vi "CameraGetData.vi"(8 "error in (no error)":errorcluster, 10 "keep open?":bool, 11 "NIvision in":refnum<class "IMAQdx.lvclass">) -> (0 "error out":errorcluster, 2 "image_data":u16[][][](array[numeric]), 3 "NIvision out":refnum<class "IMAQdx.lvclass">)   [LabVIEW 2010, in "IMAQdx.lvclass"]
uses:
  <userlib>/BIAS2/classes/IMAQdx/IMAQdx.lvclass
  <userlib>/BIAS2/classes/IMAQdx/IMAQdx.lvclass/IMAQdx.ctl
  <vilib>/vision/driver/IMAQdx.llb/IMAQdx Buffer Number Mode.ctl
  <vilib>/vision/driver/NI_Vision_Acquisition_Software.lvlib
  resource/objmgr/imaqdx.rc
  <userlib>/BIAS2/c/imaging_tools.dll
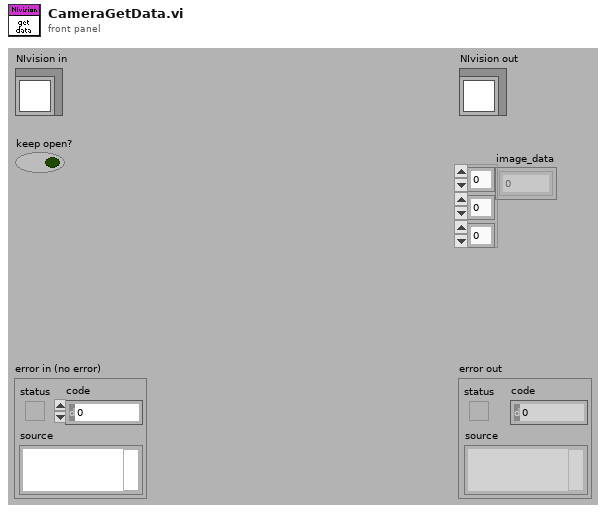
[diagram p1: front panel]
types:
  T1 = typedef "NI_Vision_Acquisition_Software.lvlib/IMAQdx Buffer Number Mode.ctl" = enum32{"Next", "Last", "Buffer Number"}
  T2 = typedef "IMAQdx.ctl" = refnum<k21>
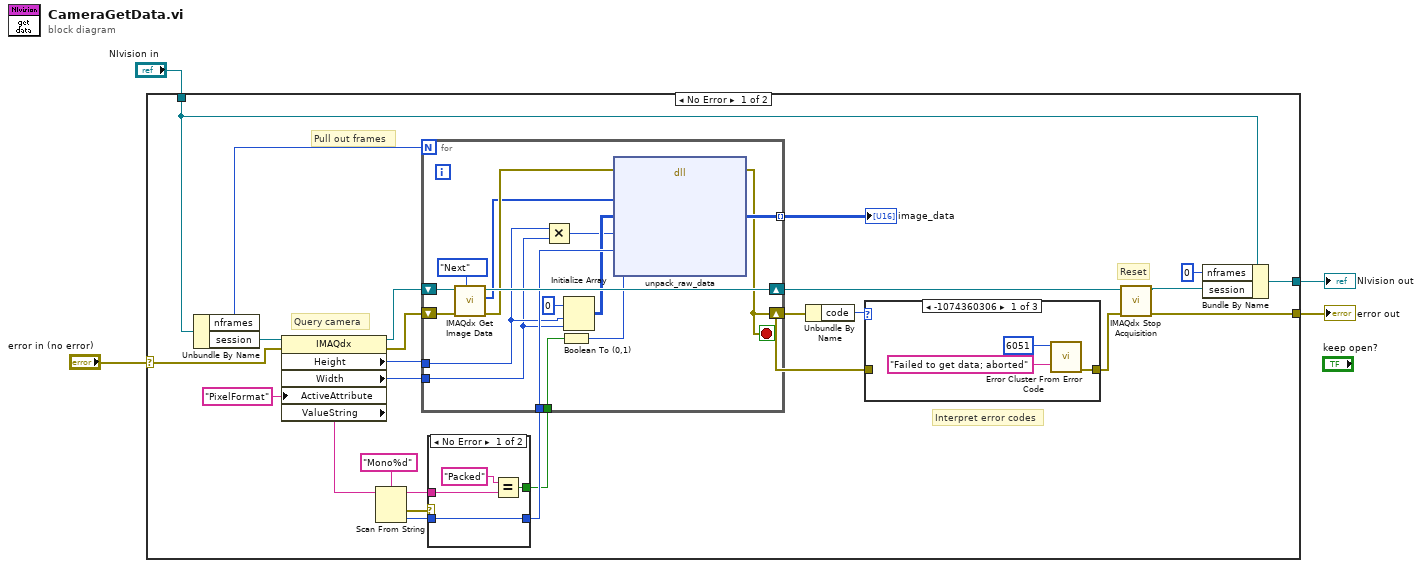
[diagram p0: block diagram]
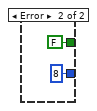
[diagram p2: hidden frame]
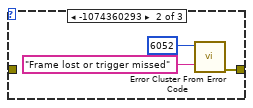
[diagram p3: hidden frame]
diagram:
  n1 = case shown="No Error" "error in (no error)" {
    selector: "error in (no error)" -> [w10 w59]
    tunnel: "NIvision in" -> [w25 w60]
    tunnel: [w9 w60] -> w2
    tunnel: [w7 w59] -> w1
    frame No Error {
      # "Query camera"
      # "Interpret error codes"
      # "Reset"
      # "Pull out frames"
      n2 = Unbundle By Name(w25) -> ("nframes"=w24:i32, "session"=w6:refnum<k21>)
      n3 = property class="IMAQdx"(reference=w6, error in=w10, "ActiveAttribute"="PixelFormat") -> (reference out=w5:refnum<k21>, error out=w28:errorcluster, "Height"=w27:u32, "Width"=w26:u32, "ValueString"=w17:string)
      n4 = Scan From String(format string="Mono%d", input string=w17) -> (remaining string=w16:string, error out=w15:errorcluster, output 1=w14:i32)  [unwired: 3 in, 1 out]
      n5 = case shown="No Error" w15 {
        tunnel: w16 -> [w33 _]
        tunnel: [w31 FALSE] -> w12
        tunnel: [w30 8] -> w13
        tunnel: w14 -> [w30 _]
        frame No Error {
          n6 = Equal?(x="Packed" ("format string"), y=w33) -> (x = y?=w31:bool)
        }
        frame Error {
        }
      }
      n7 = for {
        N: w24 -> [_]
        tunnel: [w53] -> w11 mode=indexing
        shift-right: [w57] -> w29
        shift-left: w5 -> [w58]
        shift-right: [w43] -> w21
        shift-left: w28 -> [w56]
        tunnel: w27 -> [w52]
        tunnel: w26 -> [w51]
        tunnel: w13 -> [w55]
        tunnel: w12 -> [w54]
        stop <- w43 stop-if-true
        n8 = call <vilib>:"IMAQdx Get Image Data.vi"("Buffer Number Mode (Next)"=IMAQdx_Buffer_Number_Mode."Next", "error in"=w56, "Session In"=w58) -> ("error out"=w45:errorcluster, "Image Data Array"=w44:u8[], "Session Out"=w57:T2)  [unwired: 5 in, 1 out]
        n9 = Multiply(x=w52, y=w51) -> (x*y=w47:u32)
        n10 = Boolean To (0,1)(Boolean=w54) -> (0, 1=w46:i16)
        n11 = Initialize Array(u16 0 ("element"), w52, w51) -> (w48:u16[][])
        n12 = dll-call lib="C:/Program Files/National Instruments/LabVIEW 2010/user.lib/BIAS2/c/imaging_tools.dll" fn="unpack_raw_data"(error in=w45, "in"=w44, "out"=w48, "N"=w47, "bits"=w55, "packed"=w46) -> (error out=w43:errorcluster, "out"=w53:u16[][])  [unwired: 7 in, 1 out]
      }
      "image_data" <- w11
      n13 = Unbundle By Name(w21) -> ("code"=w22:i32)
      n14 = case shown="-1074360306" w22 {
        tunnel: [w36 w39 w42] -> w20
        tunnel: w21 -> [_ _ w42]
        frame -1074360306 {
          n15 = call <vilib>:"Error Cluster From Error Code.vi"("error message (\"\")"="Failed to get data; aborted" ("error message (\"\")"), "error code (0)"=6051) -> ("error out"=w36:errorcluster)  [unwired: 7 in]
        }
        frame -1074360293 {
          n16 = call <vilib>:"Error Cluster From Error Code.vi"("error message (\"\")"="Frame lost or trigger missed" ("error message (\"\")"), "error code (0)"=6052) -> ("error out"=w39:errorcluster)  [unwired: 7 in]
        }
        frame Default {
        }
      }
      n17 = call <vilib>:"IMAQdx Stop Acquisition.vi"("error in"=w20, "Session In"=w29) -> ("error out"=w7:errorcluster, "Session Out"=w8:T2)  [unwired: 8 in]
      n18 = Bundle By Name(cluster=w25, "nframes"=0, "session"=w8) -> (w9:refnum<class "IMAQdx.lvclass">)
    }
    frame Error {
    }
  }
  "NIvision out" <- w2
  "error out" <- w1
